vi "Command Voltage Limit DAO.vi"(0 "Actuator Stroke Limit Actions":T5, 3 "Config Ref Number":T4, 7 "ID":T3, 9 "Command Voltage Limit In":T1, 11 "error in (no error)":errorcluster) -> (8 "Command Voltage Limit Out":T1, 14 "Config Ref Number out":T4, 15 "error out":errorcluster)   [LabVIEW 2009]
uses:
  Metadata/Persistant DAO Actions.ctl
  <vilib>/Utility/config.llb/Config Data RefNum.ctl
  Metadata/LBCB Number.ctl
  Metadata/Actuator Matrix.ctl
  Metadata/Actuator Point.ctl
  <vilib>/Utility/config.llb/NI_LVConfig.lvlib
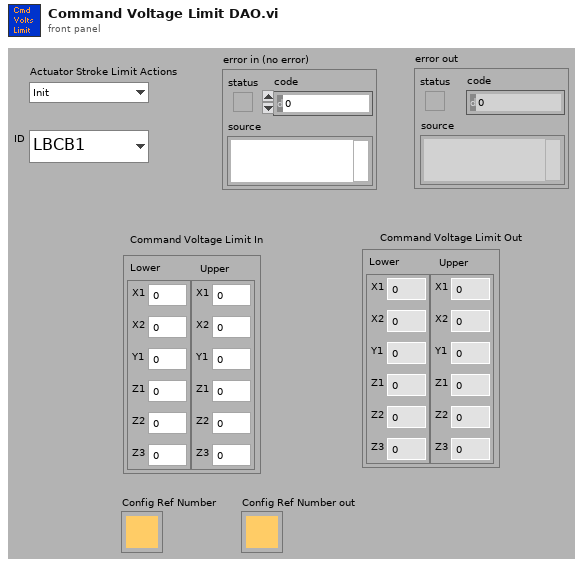
[diagram p1: front panel]
types:
  T1 = typedef "Actuator Matrix.ctl" = cluster{"Lower":T2, "Upper":T2}
  T2 = typedef "Actuator Point.ctl" = cluster{"X1":dbl, "X2":dbl, "Y1":dbl, "Z1":dbl, "Z2":dbl, "Z3":dbl}
  T3 = typedef "LBCB Number.ctl" = enum16{"LBCB1", "LBCB2"}
  T4 = typedef "NI_LVConfig.lvlib/Config Data RefNum.ctl" = refnum<k1>
  T5 = typedef "Persistant DAO Actions.ctl" = enum16{"Init", "Get", "Set", "Load", "Save"}
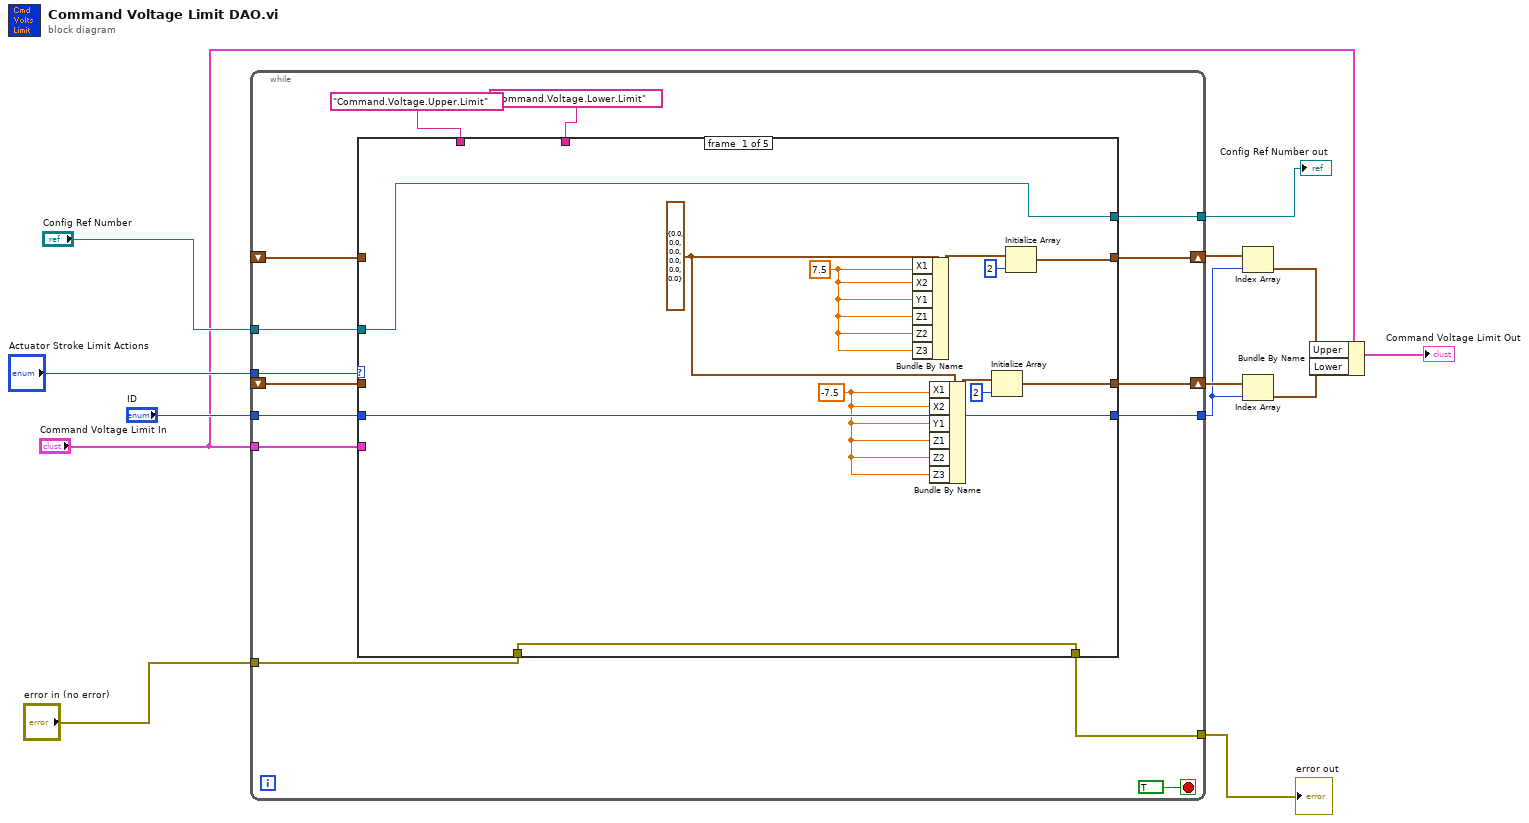
[diagram p0: block diagram]
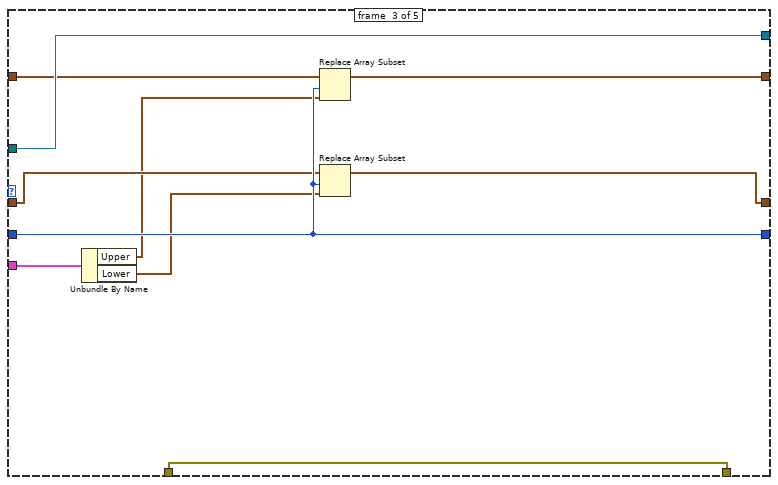
[diagram p3: hidden frame]
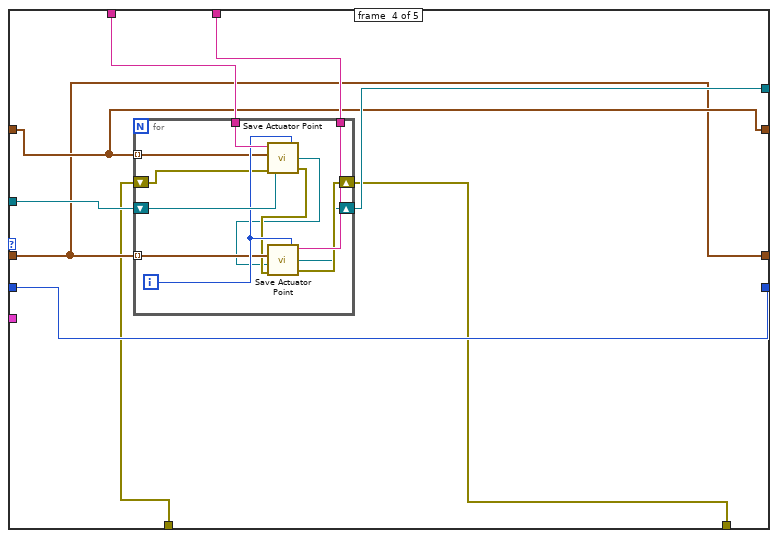
[diagram p4: hidden frame]
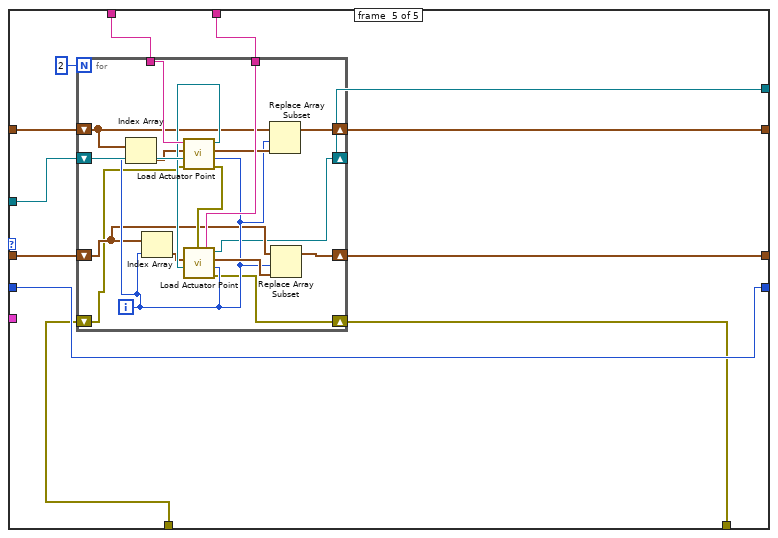
[diagram p5: hidden frame]
diagram:
  n1 = while {
    tunnel: "Actuator Stroke Limit Actions" -> [w27]
    tunnel: "Config Ref Number" -> [w26]
    tunnel: "ID" -> [w23]
    tunnel: "error in (no error)" -> [w15]
    tunnel: [w22] -> w9
    tunnel: [w21] -> w8
    tunnel: [w20] -> w5
    shift-right: [w18] -> w6
    shift-left: _ -> [w16]
    shift-right: [w19] -> w7
    shift-left: _ -> [w17]
    tunnel: "Command Voltage Limit In" -> [w14]
    stop <- TRUE stop-if-true
    n2 = case shown="\"Init\"" w27 {
      tunnel: "Command.Voltage.Upper.Limit" ("section") -> [_ _ _ w63 w86]
      tunnel: w26 -> [w40 w45 w55 w64 w87]
      tunnel: "Command.Voltage.Lower.Limit" ("section") -> [_ _ _ w62 w85]
      tunnel: w23 -> [w39 w44 w54 w60 w78]
      tunnel: [w40 w45 w55 w61 w84] -> w22
      tunnel: [w34 w41 w46 w56 w76] -> w21
      tunnel: [w39 w44 w54 w60 w78] -> w20
      tunnel: [w37 w43 w53 w59 w83] -> w19
      tunnel: [w35 w42 w52 w58 w82] -> w18
      tunnel: w17 -> [_ w43 w50 w59 w81]
      tunnel: w16 -> [_ w42 w51 w58 w80]
      tunnel: w15 -> [w34 w41 w46 w57 w77]
      tunnel: w14 -> [_ _ w49 _ _]
      frame #0 {
        w33 = T2 {"X1"=0.0, "X2"=0.0, "Y1"=0.0, "Z1"=0.0, "Z2"=0.0, "Z3"=0.0} ("Load Cell Offset In")
        w29 = -7.5 ("X1")
        w30 = 7.5 ("X1")
        n3 = Bundle By Name(cluster=w33, "X1"=w30, "X2"=w30, "Y1"=w30, "Z1"=w30, "Z2"=w30, "Z3"=w30) -> (w32:T2)
        n4 = Bundle By Name(cluster=w33, "X1"=w29, "X2"=w29, "Y1"=w29, "Z1"=w29, "Z2"=w29, "Z3"=w29) -> (w31:T2)
        n5 = Initialize Array(w31, 2 ("dimension size")) -> (w35:T2[])
        n6 = Initialize Array(w32, 2 ("dimension size")) -> (w37:T2[])
      }
      frame #1 {
      }
      frame #2 {
        n7 = Unbundle By Name(w49) -> ("Upper"=w48:T2, "Lower"=w47:T2)
        n8 = Replace Array Subset(array=w50, new element=w48, index=w54) -> (w53:T2[])
        n9 = Replace Array Subset(array=w51, new element=w47, index=w54) -> (w52:T2[])
      }
      frame #3 {
        n10 = for {
          tunnel: w63 -> [w74]
          tunnel: w62 -> [w73]
          shift-right: [w65] -> w61
          shift-left: w64 -> [w75]
          shift-right: [w67] -> w56
          shift-left: w57 -> [w69]
          tunnel: w59 -> [w71] mode=indexing
          tunnel: w58 -> [w70] mode=indexing
          i -> [w72]
          n11 = call "Save Actuator Point.vi"("LBCB Number"=w72, "error in (no error)"=w69, "refnum"=w75, "Input Cluster"=w71, "section"=w74) -> ("error out"=w68:errorcluster, "refnum out"=w66:T4)
          n12 = call "Save Actuator Point.vi"("LBCB Number"=w72, "error in (no error)"=w68, "refnum"=w66, "Input Cluster"=w70, "section"=w73) -> ("error out"=w67:errorcluster, "refnum out"=w65:T4)
        }
      }
      frame #4 {
        n13 = for {
          N: 2 -> [_]
          tunnel: w86 -> [w103]
          tunnel: w85 -> [w101]
          shift-right: [w90] -> w84
          shift-left: w87 -> [w104]
          shift-right: [w96] -> w83
          shift-left: w81 -> [w92]
          shift-right: [w95] -> w82
          shift-left: w80 -> [w91]
          shift-right: [w88] -> w76
          shift-left: w77 -> [w89]
          i -> [w97]
          n14 = Index Array(array=w92, index=w97) -> (element=w94:T2)
          n15 = Index Array(array=w91, index=w97) -> (element=w93:T2)
          n16 = call "Load Actuator Point.vi"("LBCB Number"=w97, "error in (no error)"=w89, "refnum"=w104, "Input Cluster"=w94, "section"=w103) -> ("error out"=w102:errorcluster, "Output Cluster"=w99:T2, "refnum out"=w100:T4)
          n17 = call "Load Actuator Point.vi"("LBCB Number"=w97, "error in (no error)"=w102, "refnum"=w100, "Input Cluster"=w93, "section"=w101) -> ("error out"=w88:errorcluster, "Output Cluster"=w98:T2, "refnum out"=w90:T4)
          n18 = Replace Array Subset(array=w92, new element=w99, index=w97) -> (w96:T2[])
          n19 = Replace Array Subset(array=w91, new element=w98, index=w97) -> (w95:T2[])
        }
      }
    }
  }
  "error out" <- w8
  "Config Ref Number out" <- w9
  n20 = Index Array(array=w7, index=w5) -> (element=w3:T2)
  n21 = Index Array(array=w6, index=w5) -> (element=w2:T2)
  n22 = Bundle By Name(cluster="Command Voltage Limit In", "Upper"=w3, "Lower"=w2) -> (→"Command Voltage Limit Out":T1)
